vi "load VNG captions.vi"(11 "Language Data In":T1 caption="Language Data") -> (3 "Language Data Out":T1 caption="Language Data")   [LabVIEW 2015]
uses:
  <vilib>/Utility/file.llb/Read From Spreadsheet File (string).vi
  Instance           1 25Saved   load VNG captions .vi
  Variable cluster.ctl
panel:
  out "VNG Data":T1 caption="Language Data"
  out "languages":i32
  out "all rows":string[][](array[string])
  out "first row":string[](array[string])
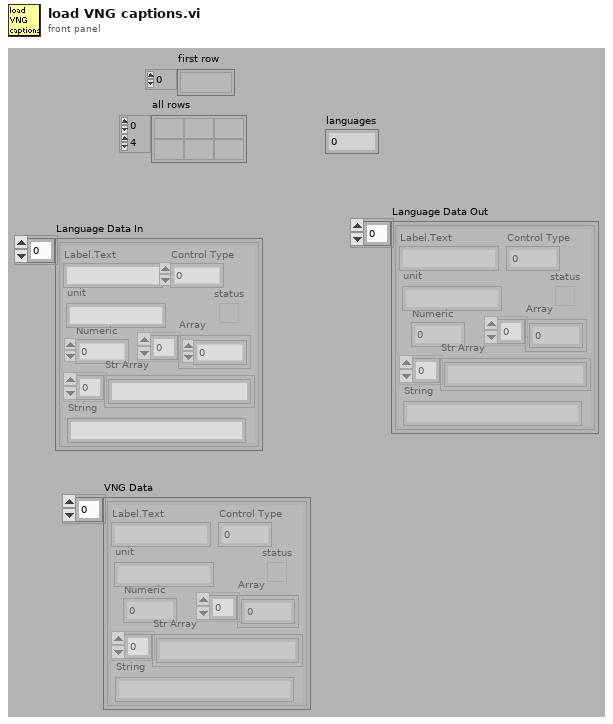
[diagram p1: front panel]
types:
  T1 = typedef "Variable cluster.ctl" = cluster{"Label.Text":string, "Control Type":u32, "Numeric":dbl, "Array":dbl[], "status":bool, "Str Array":string[], "String":string, "unit":string}[]
  T2 = cluster{"Label.Text":string, "Control Type":u32, "Numeric":dbl, "Array":dbl[], "status":bool, "Str Array":string[], "String":string, "unit":string}
  T3 = cluster{"Label.Text":string, "Control Type":u32, "Numeric":dbl, "Array":dbl[], "status":bool, "Str Array":string[], "String":string, "unit":string}[]
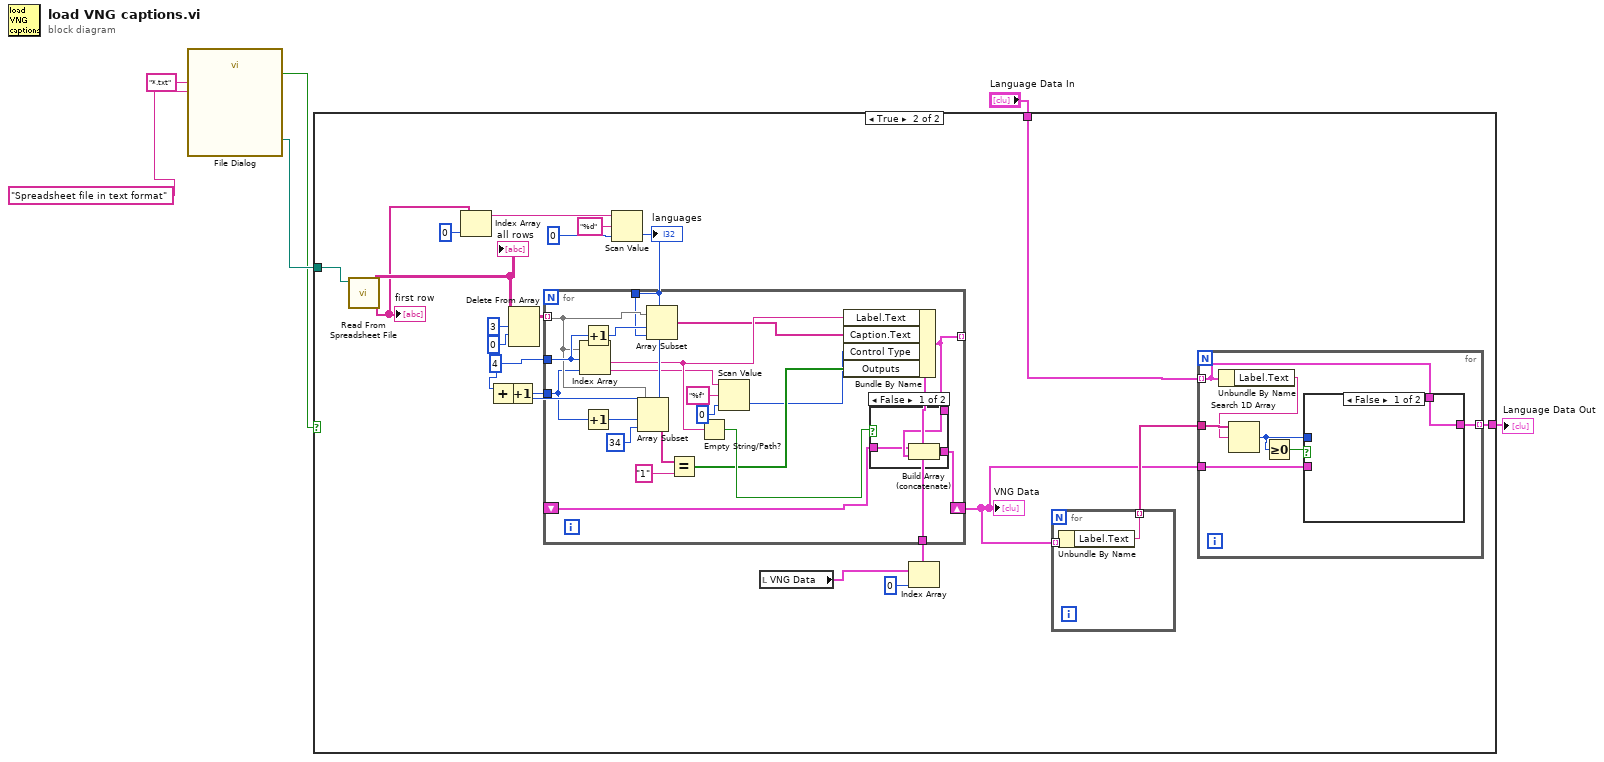
[diagram p0: block diagram]
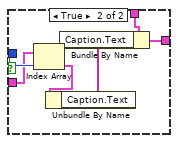
[diagram p3: hidden frame]
diagram:
  n1 = call "File Dialog"("pattern (all files)"="*.txt", "pattern label"="Spreadsheet file in text format") -> ("selected path"=w4:path, "exists"=w1:bool)  [unwired: 10 in, 2 out]
  n2 = case shown="True" w1 {
    tunnel: w4 -> [_ w13]
    tunnel: [w7 w9] -> w3
    tunnel: "Language Data In" -> [w7 w8]
    frame False {
    }
    frame True {
      w18 = 4 ("index")
      n3 = call-poly <vilib>:"Read From Spreadsheet File.vi"("file path (dialog if empty)"=w13) -> ("first row"=w23:string[], "all rows"=w28:string[][])  [unwired: 6 in, 3 out]
      "first row" <- w23
      "all rows" <- w28
      n4 = Index Array(array=w23, index=0) -> (element=w21:string)
      n5 = Delete From Array(array=w28, length=3, index (row)=0) -> (array with subset deleted=w25:string[][])  [unwired: 1 in, 1 out]
      n6 = Scan Value(string=w21, format string="%d", default (0 dbl)=0) -> (value=w17:i32)  [unwired: 1 out]
      "languages" <- w17
      n7 = Add(x=w18, y=w17) -> (x+y=w19:i32)
      n8 = Increment(x=w19) -> (x+1=w16:i32)
      n9 = local read "VNG Data"() -> (w12:T1)
      n10 = Index Array(array=w12, index=0) -> (element=w14:T2)
      n11 = for {
        tunnel: w25 -> [w54] mode=indexing
        tunnel: [w61] -> _ mode=indexing
        shift-right: [w65] -> w10
        shift-left: _ -> [w56]
        tunnel: w18 -> [w58]
        tunnel: w16 -> [w48]
        tunnel: w17 -> [w49]
        tunnel: w14 -> [w55]
        n12 = Index Array(array=w54, index #1=w58, index #2=w48) -> (element #1=w63:string, element #2=w60:string)
        n13 = Increment(x=w58) -> (x+1=w57:i32)
        n14 = Increment(x=w48) -> (x+1=w47:i32)
        n15 = Array Subset(array=w54, index=w47, length=34) -> (w52:string[])
        n16 = Array Subset(array=w54, index=w57, length=w49) -> (w59:string[])
        n17 = Equal?(x=w52, y="1") -> (x = y?=w50:bool[])
        n18 = Empty String/Path?(string/path=w63) -> (empty?=w62:bool)
        n19 = Scan Value(string=w60, format string="%f", default (0 dbl)=u32 0 ("Control Type")) -> (value=w46:u32)  [unwired: 1 out]
        n20 = Bundle By Name(cluster=w55, "Label.Text"=w63, "Caption.Text"=w59, "Control Type"=w46, "Outputs"=w50) -> (w61:T2)
        n21 = case shown="False" w62 {
          tunnel: w61 -> [w68 _]
          tunnel: w56 -> [w67 w69]
          tunnel: [w66 w69] -> w65
          frame False {
            n22 = Build Array (concatenate)(w67, w68) -> (w66:T3)
          }
          frame True {
          }
        }
      }
      "VNG Data" <- w10
      n23 = for {
        tunnel: w10 -> [w30] mode=indexing
        tunnel: [w29] -> w11 mode=indexing
        n24 = Unbundle By Name(w30) -> ("Label.Text"=w29:string)
      }
      n25 = for {
        tunnel: w8 -> [w34] mode=indexing
        tunnel: w11 -> [w37]
        tunnel: w10 -> [w35]
        tunnel: [w33] -> w9 mode=indexing
        n26 = Unbundle By Name(w34) -> ("Label.Text"=w36:string)
        n27 = Search 1D Array(1D array=w37, element=w36) -> (index of element=w31:i32)  [unwired: 1 in]
        n28 = Greater Or Equal To 0?(x=w31) -> (x >= 0?=w32:bool)
        n29 = case shown="False" w32 {
          tunnel: w31 -> [_ w44]
          tunnel: w35 -> [_ w43]
          tunnel: w34 -> [w38 w42]
          tunnel: [w38 w39] -> w33
          frame False {
          }
          frame True {
            n30 = Index Array(array=w43, index=w44) -> (element=w41:T2)
            n31 = Unbundle By Name(w41) -> ("Caption.Text"=w40:string[])
            n32 = Bundle By Name(cluster=w42, "Caption.Text"=w40) -> (w39:T2)
          }
        }
      }
    }
  }
  "Language Data Out" <- w3
